vi "Rotate Data By Teeth Angle.vi"(5 "Position reference":T1 caption="FPGA simulation angle reference", 7 "Missing Tooth Angle":dbl, 11 "One VR Crank Period":dbl[](array[numeric])) -> (3 "Rotated to desired angle":dbl[](array[numeric]))   [LabVIEW 2013, in "Engine Simulation Toolkit System Explorer.lvlib"]
uses:
  Engine Simulation Toolkit System Explorer.lvlib
  Position Reference.ctl
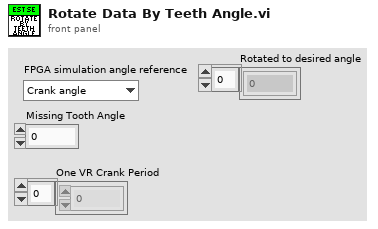
[diagram p1: front panel]
types:
  T1 = typedef "Engine Simulation Toolkit System Explorer.lvlib/Position Reference.ctl" = enum16{"Crank angle", "Cycle angle"}
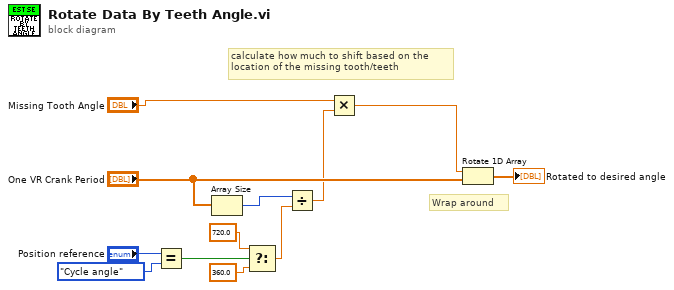
[diagram p0: block diagram]
diagram:
  # "Wrap around"
  # "calculate how much to shift based on the \nlocation of the missing tooth/teeth"
  n1 = Equal?(x="Position reference", y=Position_Reference."Cycle angle") -> (x = y?=w1:bool)
  n2 = Array Size(array="One VR Crank Period") -> (size(s)=w7:i32)
  n3 = Select(t=720.0, s=w1, f=360.0 ("t")) -> (s? t:f=w4:dbl)
  n4 = Divide(x=w7, y=w4) -> (x/y=w9:dbl)
  n5 = Multiply(x="Missing Tooth Angle", y=w9) -> (x*y=w10:dbl)
  n6 = Rotate 1D Array(1:"One VR Crank Period", 2:w10) -> (0:→"Rotated to desired angle":dbl[])
